vi "Logger.handleFileContent.vi"(11 "ResultsFile":dbl[](array[numeric]) format="%#_6f") -> (3 "HandledFileContent":T1 {"Values" format="%.3f"})   [LabVIEW 2016]
uses:
  Logger.FileBody.ctl
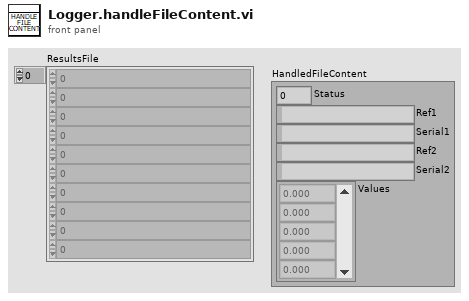
[diagram p1: front panel]
types:
  T1 = typedef "Logger.FileBody.ctl" = cluster{"Status":u8, "Ref1":string, "Serial1":string, "Ref2":string, "Serial2":string, "Values":sgl[]}
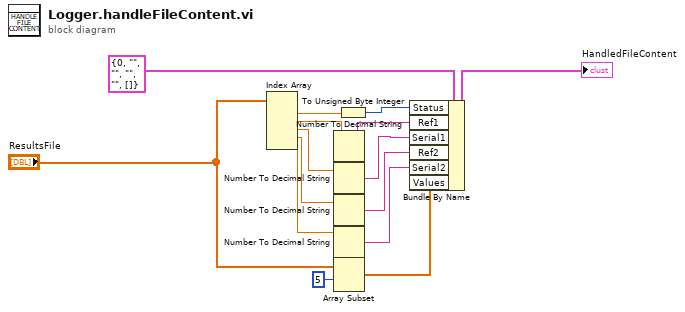
[diagram p0: block diagram]
diagram:
  n1 = Index Array(array="ResultsFile") -> (element #1=w1:dbl, element #2=w12:dbl, element #3=w9:dbl, element #4=w8:dbl, element #5=w7:dbl)  [unwired: 5 in]
  n2 = Number To Decimal String(number=w12) -> (decimal integer string=w11:string)  [unwired: 1 in]
  n3 = Number To Decimal String(number=w9) -> (decimal integer string=w10:string)  [unwired: 1 in]
  n4 = Number To Decimal String(number=w8) -> (decimal integer string=w6:string)  [unwired: 1 in]
  n5 = Number To Decimal String(number=w7) -> (decimal integer string=w5:string)  [unwired: 1 in]
  n6 = Array Subset(array="ResultsFile", index=5) -> (w3:dbl[])  [unwired: 1 in]
  n7 = To Unsigned Byte Integer(number=w1) -> (unsigned 8bit integer=w2:u8)
  n8 = Bundle By Name(cluster=T1 {"Status"=0, "Ref1"="", "Serial1"="", "Ref2"="", "Serial2"="", "Values"=[]} ("PLCvalues"), "Status"=w2, "Ref1"=w11, "Serial1"=w10, "Ref2"=w6, "Serial2"=w5, "Values"=w3) -> (→"HandledFileContent":T1)
